vi "Save Process to Library.vi"(8 "Error In":errorcluster, 9 "Process":string, 10 "Library Path":path, 11 "CS++DSCManager in":refnum<class "CS++DSCManager.lvclass">) -> (0 "Error Out":errorcluster, 2 "Complete Path":path, 3 "CS++DSCManager out":refnum<class "CS++DSCManager.lvclass">)   [LabVIEW 2016, in "CS++DSCManager.lvlib" / "CS++DSCManager.lvclass"]
doc: "Saves the deployed configuration of processes or shared variables to one or several LabVIEW project libraries."
uses:
  CS++DSCManager.lvclass
  <vilib>/lvdsc/process/ProcessToLib.vi
  <vilib>/lvdsc/NI_DSC.lvlib
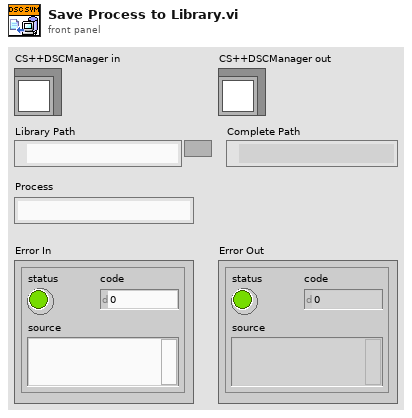
[diagram p1: front panel]
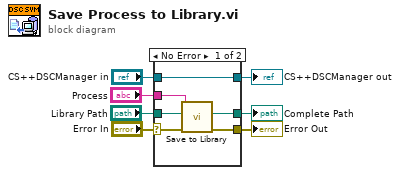
[diagram p0: block diagram]
diagram:
  n1 = case shown="No Error" "Error In" {
    selector: "Error In" -> [w13 w16]
    tunnel: [w9 w16] -> w2
    tunnel: [w10 w15] -> w5
    tunnel: "CS++DSCManager in" -> [w10 w15]
    tunnel: "Library Path" -> [w12 w14]
    tunnel: "Process" -> [w11 _]
    tunnel: [w8 w14] -> w1
    frame No Error {
      n2 = call-poly <vilib>:"Save to Library.vi"("error in (no error)"=w13, "library path"=w12, "process"=w11) -> ("error out"=w9:errorcluster, "complete path"=w8:path)  [unwired: 7 in]
    }
    frame Error {
    }
  }
  "Error Out" <- w2
  "CS++DSCManager out" <- w5
  "Complete Path" <- w1
